vi "YKMW100 Send Querry Recieve Message.vi"(0 "VISA session":refnum<visa-resource-name>="MW100", 7 "Send Message (\"\")":string, 9 "Timeout (25000)":u32=100, 11 "error in (no error)":errorcluster, 13 "Source (\"\")":string) -> (4 "dup VISA session":refnum<visa-resource-name>, 8 "Read Buffer":string, 15 "error out":errorcluster)   [LabVIEW 2009]
doc: "This VI sends the message. Then it returns the response."
panel:
  out "ENCRLF":string
  out "EACRLF":string
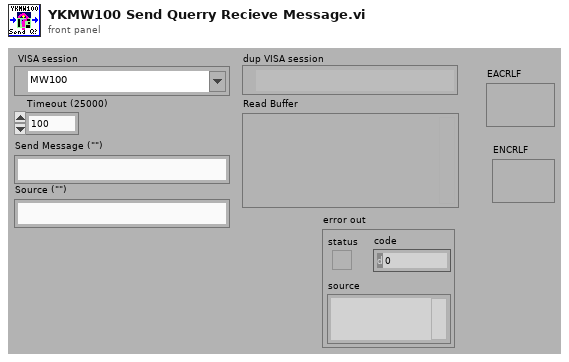
[diagram p1: front panel]
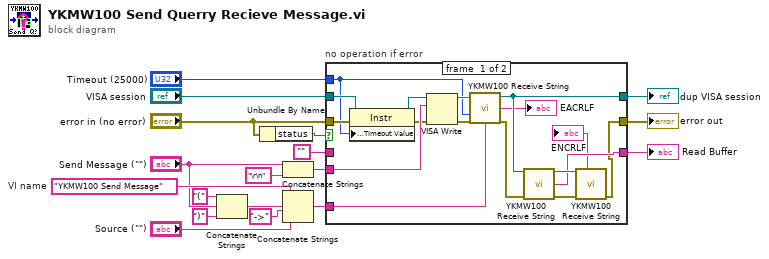
[diagram p0: block diagram]
diagram:
  w6 = "YKMW100 Send Message"  # VI name
  n1 = Concatenate Strings("(", "Send Message (\"\")", ")") -> (w7:string)
  n2 = Unbundle By Name("error in (no error)") -> ("status"=w13:bool)
  n3 = Concatenate Strings("Send Message (\"\")", "\r\n") -> (w17:string)
  n4 = Concatenate Strings(w6, w7, "->", "Source (\"\")") -> (w12:string)
  n5 = case "no operation if error" shown="False" w13 {
    tunnel: "VISA session" -> [w32 w38]
    tunnel: w17 -> [w35 _]
    tunnel: [w24 w38] -> w4
    tunnel: [w21 w37] -> w18
    tunnel: "error in (no error)" -> [w34 w37]
    tunnel: w12 -> [w28 _]
    tunnel: "Timeout (25000)" -> [w27 _]
    tunnel: [w22 w36] -> w5
    tunnel: "" -> [_ w36]
    frame #0 {
      n6 = property class="Instr"(reference=w32, error in=w34, "General Settings:Timeout Value"=w27) -> (reference out=w31:refnum<visa-resource-name>, error out=w33:errorcluster)
      n7 = VISA Write(VISA resource name=w31, write buffer=w35, error in (no error)=w33) -> (VISA resource name out=w30:refnum<visa-resource-name>, error out=w29:errorcluster)  [unwired: 1 out]
      n8 = call "YKMW100 Receive String.vi"("VISA session"=w30, "Timeout (25000)"=w27, "error in (no error)"=w29, "Source (\"\")"=w28) -> ("dup VISA session"=w24:refnum<visa-resource-name>, "Read Buffer"=→"EACRLF":string, "error out"=w23:errorcluster)  [unwired: 9 in]
      n9 = call "YKMW100 Receive String.vi"("VISA session"=w24, "error in (no error)"=w23) -> ("dup VISA session"=w26:refnum<visa-resource-name>, "Read Buffer"=w22:string, "error out"=w25:errorcluster)  [unwired: 11 in]
      n10 = call "YKMW100 Receive String.vi"("VISA session"=w26, "error in (no error)"=w25) -> ("Read Buffer"=→"ENCRLF":string, "error out"=w21:errorcluster)  [unwired: 11 in, 1 out]
    }
    frame #1 {
    }
  }
  "error out" <- w18
  "dup VISA session" <- w4
  "Read Buffer" <- w5
